vi "Is Initialized.vi"(8 "error in":errorcluster, 11 "IInitialize in":refnum<class "IInitialize.lvclass">) -> (0 "error out":errorcluster, 2 "Is Initialized?":bool, 3 "IInitialize out":refnum<class "IInitialize.lvclass">)   [LabVIEW 2024, in "IInitialize.lvclass"]
uses:
  IInitialize.lvclass
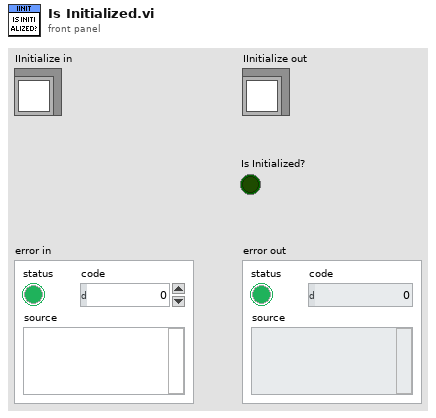
[diagram p1: front panel]
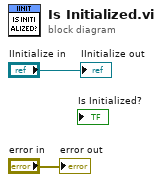
[diagram p0: block diagram]
diagram:
  "IInitialize out" <- "IInitialize in"
  "error out" <- "error in"
